vi "Capacitance Estimator.vi"(0 "Resistance (Ohms)":dbl=100000.0 format="%.4e", 11 "normalized waveform":waveform(dbl)={"t0"=timestamp(3087922235.213 s since 1904-01-01), "dt"=1.9999999494757503e-05, "Y"=array[1000 elements]}) -> (4 "Estimated Capacitance (F)":dbl format="%.4e", 15 "time constant (s)":dbl)   [LabVIEW 2019]
doc: "This is a Bug C(T) subVI.\n\nGiven an RC decay waveform and the resistance R, this vi estimates the capacitance by determining the 1/e time.\n\nPaul K Dixon\nPhysics 3600\nCSUSB Physics"
panel:
  # "C(T) Capacitance Estimator"
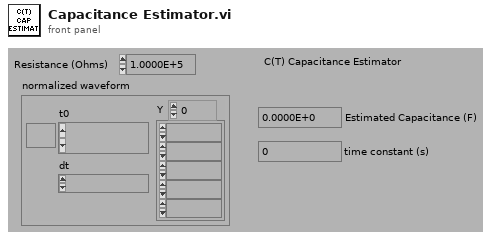
[diagram p1: front panel]
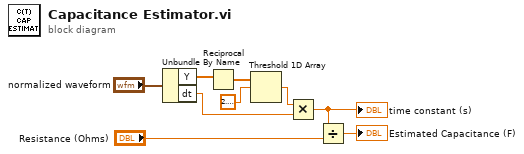
[diagram p0: block diagram]
diagram:
  n1 = Unbundle By Name("normalized waveform") -> ("Y"=w8:dbl[], "dt"=w4:dbl)
  n2 = Reciprocal(x=w8) -> (1/x=w7:dbl[])
  n3 = Threshold 1D Array(2:2.718281828459045, 3:w7) -> (0:w5:dbl)  [unwired: 1 out]
  n4 = Multiply(x=w5, y=w4) -> (x*y=w3:dbl)
  "time constant (s)" <- w3
  n5 = Divide(x=w3, y="Resistance (Ohms)") -> (x/y=→"Estimated Capacitance (F)":dbl)
